vi "Read Open Thermocouple Detection.vi"(8 "error in":errorcluster, 11 "NI 9213 in":refnum<class "NI 9213.lvclass">) -> (0 "error out":errorcluster, 2 "open thermocouple detection":bool, 3 "NI 9213 out":refnum<class "NI 9213.lvclass">)   [LabVIEW 2017, in "Scan Engine Scripting.lvlib" / "NI 9213.lvclass"]
doc: "Reads the open thermocouple detection from the module private data."
uses:
  NI 9213.lvclass
  NI 9213.lvclass/NI 9213.ctl
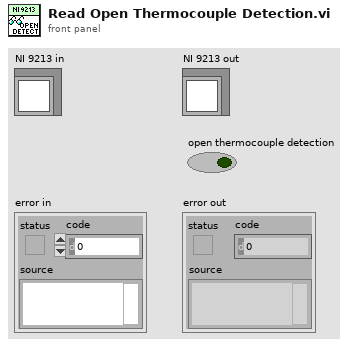
[diagram p1: front panel]
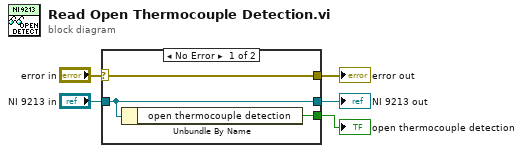
[diagram p0: block diagram]
diagram:
  n1 = case shown="No Error" "error in" {
    selector: "error in" -> [w8 w9]
    tunnel: [w8 w9] -> w4
    tunnel: [w7 w10] -> w1
    tunnel: "NI 9213 in" -> [w7 w10]
    tunnel: [w6 _] -> w3
    frame No Error {
      n2 = Unbundle By Name(w7) -> ("open thermocouple detection"=w6:bool)
    }
    frame Error {
    }
  }
  "error out" <- w4
  "open thermocouple detection" <- w3
  "NI 9213 out" <- w1
